vi "Write JSON properties.vi"(8 "error in (no error)":errorcluster, 10 "UI VI ref":refnum<vi>, 11 "ZenGage v3.0 UI in":refnum<class "ZenGage v3.0 UI.lvclass">) -> (0 "error out":errorcluster, 3 "ZenGage v3.0 UI out":refnum<class "ZenGage v3.0 UI.lvclass">)   [LabVIEW 2015, in "ZenGage v3.0 UI.lvclass"]
uses:
  ZenGage v3.0 UI.lvclass
  <vilib>/Utility/miscctls.llb/LVRectTypeDef.ctl
  ZenGage v3.0 UI.lvclass/ZenGage v3.0 UI.ctl
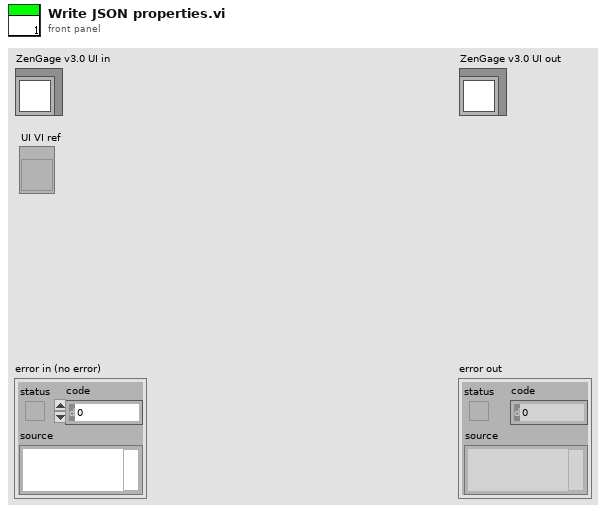
[diagram p1: front panel]
types:
  T1 = typedef "LVRectTypeDef.ctl" = cluster{"Left":i16, "Top":i16, "Right":i16, "Bottom":i16}
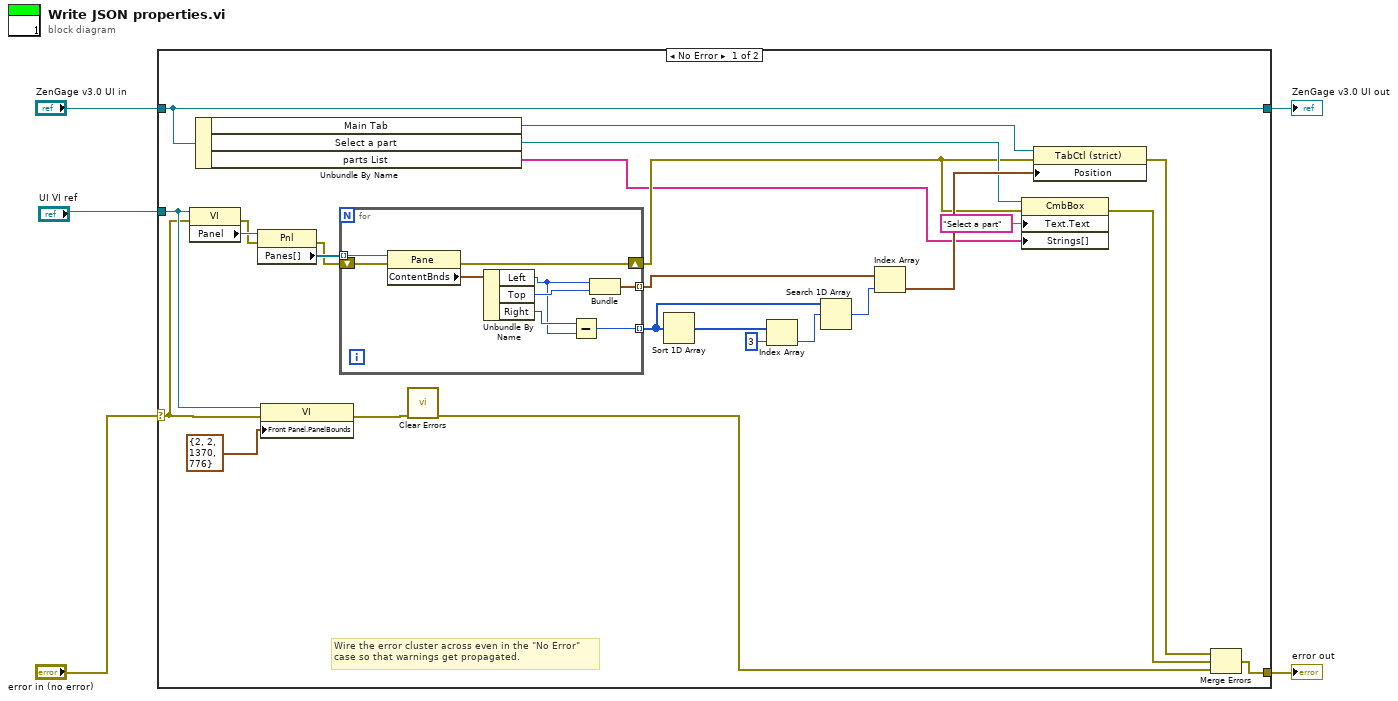
[diagram p0: block diagram]
diagram:
  n1 = case shown="No Error" "error in (no error)" {
    selector: "error in (no error)" -> [w16 w41]
    tunnel: [w17 w41] -> w4
    tunnel: [w30 w40] -> w2
    tunnel: "ZenGage v3.0 UI in" -> [w30 w40]
    tunnel: "UI VI ref" -> [w19 _]
    frame No Error {
      # "Wire the error cluster across even in the \"No Error\"\ncase so that warnings get propagated."
      n2 = property class="VI"(reference=w19, error in=w16) -> (error out=w15:errorcluster, "Panel"=w20:refnum<vi>)  [unwired: 1 out]
      n3 = Unbundle By Name(w30) -> ("Main Tab"=w29:refnum<vi>, "Select a part"=w11:refnum<vi>, "parts List"=w7:string[])
      n4 = property class="Pnl"(reference=w20, error in=w15) -> (error out=w14:errorcluster, "Panes[]"=w28:refnum<vi>[])  [unwired: 1 out]
      n5 = property class="VI"(reference=w19, error in=w16, "Front Panel.PanelBounds"=T1 {"Left"=2, "Top"=2, "Right"=1370, "Bottom"=776} ("Front Panel Window:Panel Bounds")) -> (error out=w13:errorcluster)  [unwired: 1 out]
      n6 = for {
        tunnel: w28 -> [w39] mode=indexing
        tunnel: [w36] -> w23 mode=indexing
        tunnel: [w33] -> w25 mode=indexing
        shift-right: [w31] -> w10
        shift-left: w14 -> [w32]
        n7 = property class="Pane"(reference=w39, error in=w32) -> (error out=w31:errorcluster, "ContentBnds"=w38:T1)  [unwired: 1 out]
        n8 = Unbundle By Name(w38) -> ("Left"=w34:i16, "Top"=w37:i16, "Right"=w35:i16)
        n9 = Subtract(x=w35, y=w34) -> (x-y=w33:i16)
        n10 = Bundle("Left"=w34, "Top"=w37) -> (w36:cluster{"Left":i16, "Top":i16})  [unwired: 1 in]
      }
      n11 = call <vilib>:"Clear Errors.vi"("error in (no error)"=w13) -> ("error out"=w12:errorcluster)  [unwired: 5 in, 1 out]
      n12 = Sort 1D Array(array=w25) -> (sorted array=w27:i16[])
      n13 = Index Array(array=w27, index=3) -> (element=w24:i16)
      n14 = Search 1D Array(1D array=w25, element=w24) -> (index of element=w22:i32)  [unwired: 1 in]
      n15 = Index Array(array=w23, index=w22) -> (element=w21:cluster{"Left":i16, "Top":i16})
      n16 = property class="CmbBox"(reference=w11, error in=w10, "Text.Text"="Select a part", "Strings[]"=w7) -> (error out=w8:errorcluster)  [unwired: 1 out]
      n17 = property class="TabCtl (strict)"(reference=w29, error in=w10, "Position"=w21) -> (error out=w9:errorcluster)  [unwired: 1 out]
      n18 = Merge Errors(w9, w8, w12) -> (w17:errorcluster)
    }
    frame Error {
    }
  }
  "error out" <- w4
  "ZenGage v3.0 UI out" <- w2
